vi "Periodic Tasks.vi"(8 "error in":errorcluster) -> ()   [LabVIEW 2018]
doc: "This VI runs in parallel to other tasks. It can contain as many user-defined periodic loops as you need. These can carry out PID or other sorts of timed response."
uses:
  <vilib>/Rock Robotics/WPI/ThirdParty/Phoenix-LabVIEW/Motor Controller/Controls/CTRE_Phoenix_MotorControl_ControlMode.ctl
  <vilib>/Rock Robotics/WPI/Solenoid/WPI_SolenoidValue.ctl
  <vilib>/Rock Robotics/WPI/Utilities/WPI_GetSetVariantRefNum.vi
  Robot Global Data.vi
  <vilib>/Rock Robotics/WPI/Solenoid/WPI_SolenoidSetEnum.vi
  <vilib>/Rock Robotics/WPI/RobotDrive/WPI_RobotDriveArcadeDrive_Standard(NoSaturation).vi
  <vilib>/Rock Robotics/WPI/ThirdParty/Phoenix-LabVIEW/Motor Controller/Get/CTRE_Phoenix_MotorController_GetQuadratureData.vi
panel:
  out "Waveform Chart":T1(graph)
  in  "Zero":bool
  out "Quadrature Position 2":i32
  out "Quadrature Position":i32
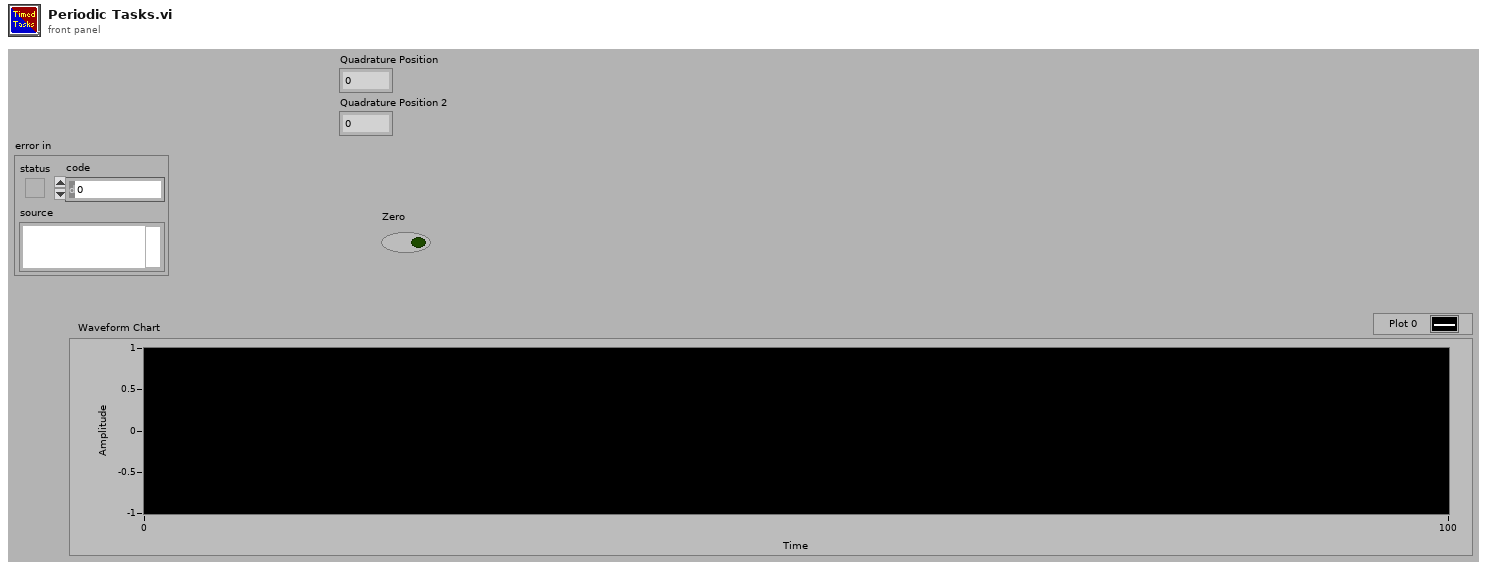
[diagram p1: front panel]
types:
  T1 = cluster{"Quadrature Position":i32, "Quadrature Position":i32}
  T2 = typedef "WPI_MotorControlDeviceRef.ctl" = cluster{"DeviceStatus":errorcluster, "Type":T3, "PWM":cluster{"PWM Channel":T4, "DeadBand":T5}, "CAN":cluster{"Device Number":u8, "SetOutput VI Ref":variant, "GetOutput VI Ref":variant, "Enable VI Ref":variant, "Disable VI Ref":variant, "Data":variant}, "Invert":bool, "DIO PWM":cluster{"PWM \"Enable\" Channel":T4, "DIOChannel":T6, "PWM Rate":dbl}}
  T3 = typedef "WPI_MotorControlType.ctl" = enum16{"PWM", "CAN", "DIO PWM"}
  T4 = typedef "FPGA_DIOPWMChannel.ctl" = enum8{"PWM 0", "PWM 1", "PWM 2", "PWM 3", "PWM 4", "PWM 5", "PWM 6", "PWM 7", "PWM 8", "PWM 9", "PWM MXP 0", "PWM MXP 1", "PWM MXP 2", "PWM MXP 3", "PWM MXP 4", "PWM MXP 5", "PWM MXP 6", "PWM MXP 7", "PWM MXP 8", "PWM MXP 9", "Invalid"}
  T5 = typedef "WPI_PWMDeadband.ctl" = cluster{"Name":string, "maxPositivePwm":i32, "minPositivePwm":i32, "centerPwm":i32, "maxNegativePwm":i32, "minNegativePwm":i32, "angularRange":u16}
  T6 = typedef "FPGA_DIOChannel.ctl" = enum8{"DIO 0", "DIO 1", "DIO 2", "DIO 3", "DIO 4", "DIO 5", "DIO 6", "DIO 7", "DIO 8", "DIO 9", "DIO MXP 0", "DIO MXP 1", "DIO MXP 2", "DIO MXP 3", "DIO MXP 4", "DIO MXP 5", "DIO MXP 6", "DIO MXP 7", "DIO MXP 8", "DIO MXP 9", "DIO MXP 10", "DIO MXP 11", "DIO MXP 12", "DIO MXP 13", "DIO MXP 14", "DIO MXP 15", "SPI Port CS1", "SPI Port CS2", "SPI Port CS3", "SPI Port MISO", "SPI Port MOSI", "Invalid"}
  T7 = typedef "WPI_JoystickDevRef.ctl" = cluster{"Device":T8}
  T8 = typedef "WPI_JoystickDeviceEnum.ctl" = enum16{"USB 0", "USB 1", "USB 2", "USB 3", "USB 4", "USB 5"}
  T9 = typedef "WPI_RobotDriveDevRef.ctl" = cluster{"DevStatus":errorcluster, "Motors[]":T2[], "Square Inputs":bool, "Max Output":dbl}
  T10 = typedef "WPI_SolenoidDevRef.ctl" = cluster{"DevStatus":errorcluster, "Pneumatics Control Module":u8, "Forward Solenoid Channel":T11, "Reverse Solenoid Channel":T11}
  T11 = typedef "WPI_SolenoidChannel.ctl" = enum8{"Solenoid 0", "Solenoid 1", "Solenoid 2", "Solenoid 3", "Solenoid 4", "Solenoid 5", "Solenoid 6", "Solenoid 7", "Invalid"}
  T12 = typedef "WPI_SolenoidValue.ctl" = enum16{"Off", "On", "Forward", "Reverse"}
  T13 = typedef "CTRE_Phoenix_MotorControl_ControlMode.ctl" = u16
  T14 = typedef "WPI_DriverStationRobotMode2.ctl" = enum16{"Autonomous Disabled", "Autonomous Enabled", "Teleop Disabled", "Teleop Enabled", "Disconnected", "Finish", "Test Disabled", "Test Enabled", "Emergency Stopped"}
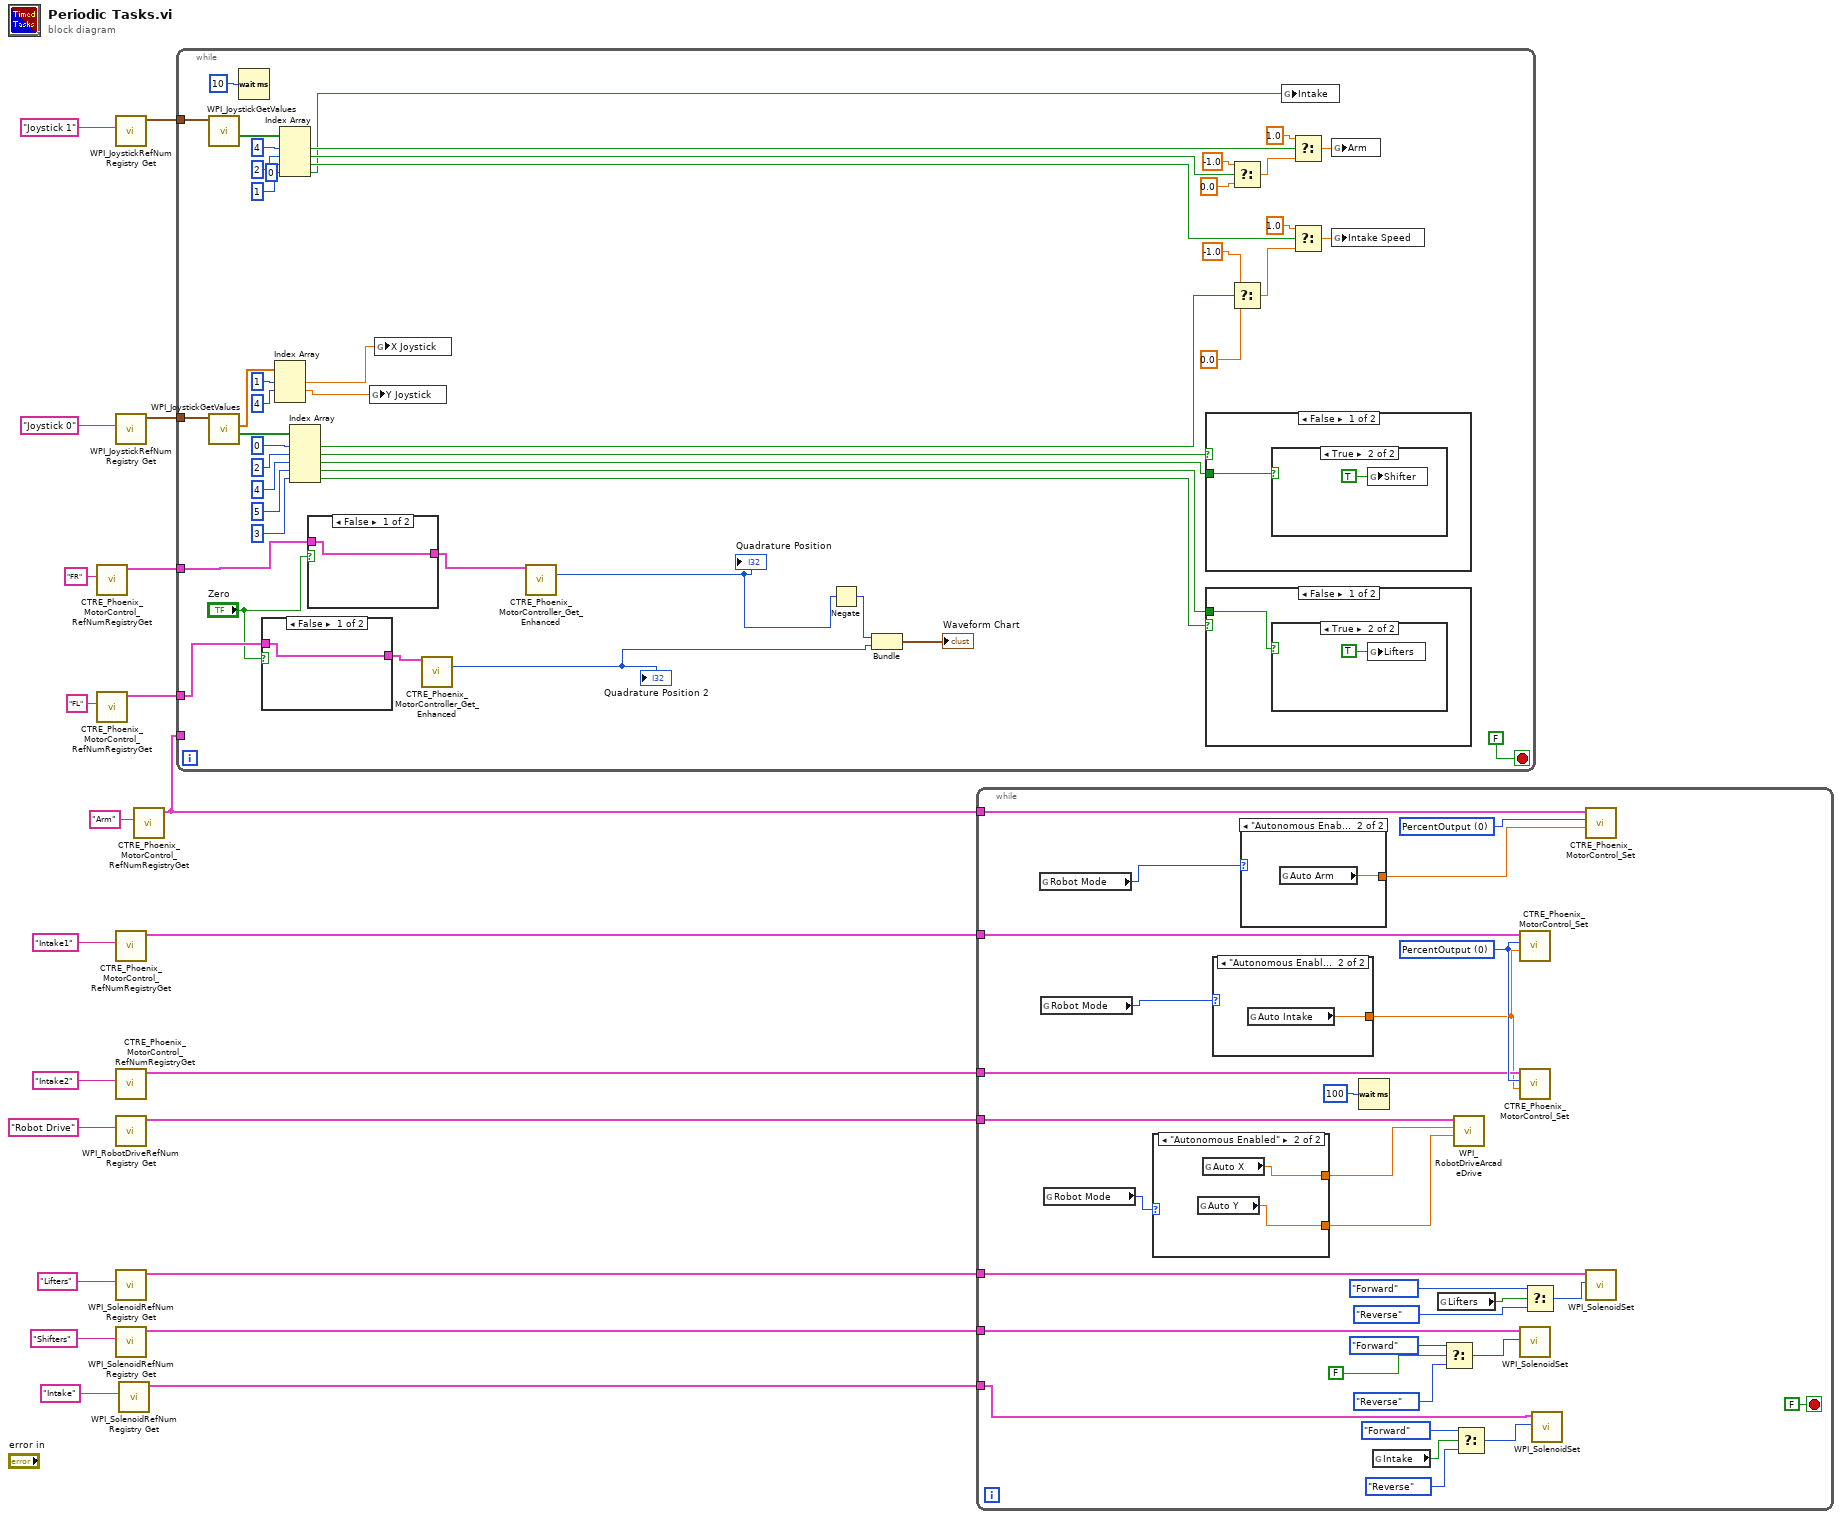
[diagram p0: block diagram]
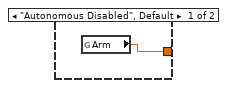
[diagram p2: hidden frame]
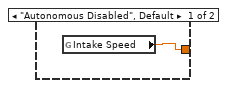
[diagram p3: hidden frame]
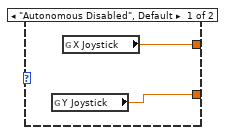
[diagram p4: hidden frame]
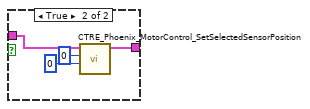
[diagram p5: hidden frame]
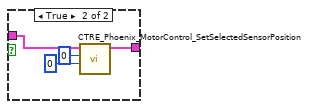
[diagram p6: hidden frame]
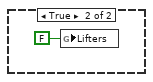
[diagram p8: hidden frame]
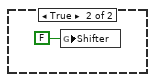
[diagram p10: hidden frame]
diagram:
  n1 = call <vilib>:"CTRE_Phoenix_MotorControl_RefNumRegistryGet.vi"("refnum name"="FR") -> ("PhoenixMotorControlDevRef"=w2:T2)  [unwired: 9 in, 1 out]
  n2 = call <vilib>:"CTRE_Phoenix_MotorControl_RefNumRegistryGet.vi"("refnum name"="FL") -> ("PhoenixMotorControlDevRef"=w1:T2)  [unwired: 9 in, 1 out]
  n3 = call <vilib>:"WPI_JoystickRefNum Registry Get.vi"("refnum name"="Joystick 1") -> ("JoystickDevRef"=w16:T7)  [unwired: 1 in, 9 out]
  n4 = call <vilib>:"WPI_JoystickRefNum Registry Get.vi"("refnum name"="Joystick 0") -> ("JoystickDevRef"=w15:T7)  [unwired: 1 in, 9 out]
  n5 = call <vilib>:"CTRE_Phoenix_MotorControl_RefNumRegistryGet.vi"("refnum name"="Intake1") -> ("PhoenixMotorControlDevRef"=w14:T2)  [unwired: 9 in, 1 out]
  n6 = call <vilib>:"CTRE_Phoenix_MotorControl_RefNumRegistryGet.vi"("refnum name"="Intake2") -> ("PhoenixMotorControlDevRef"=w13:T2)  [unwired: 9 in, 1 out]
  n7 = call <vilib>:"WPI_RobotDriveRefNum Registry Get.vi"("refnum name"="Robot Drive") -> ("RobotDriveDevRef"=w12:T9)  [unwired: 1 in, 9 out]
  n8 = call <vilib>:"WPI_SolenoidRefNum Registry Get.vi"("refnum name"="Lifters") -> ("SolenoidDevRef"=w7:T10)  [unwired: 9 in, 1 out]
  n9 = call <vilib>:"WPI_SolenoidRefNum Registry Get.vi"("refnum name"="Shifters") -> ("SolenoidDevRef"=w9:T10)  [unwired: 9 in, 1 out]
  n10 = call <vilib>:"WPI_SolenoidRefNum Registry Get.vi"("refnum name"="Intake") -> ("SolenoidDevRef"=w5:T10)  [unwired: 9 in, 1 out]
  n11 = call <vilib>:"CTRE_Phoenix_MotorControl_RefNumRegistryGet.vi"("refnum name"="Arm") -> ("PhoenixMotorControlDevRef"=w11:T2)  [unwired: 9 in, 1 out]
  n12 = while {
    tunnel: w16 -> [w55]
    tunnel: w15 -> [w56]
    tunnel: w11 -> [_]
    tunnel: w2 -> [w31]
    tunnel: w1 -> [w33]
    stop <- FALSE stop-if-true
    n13 = call <vilib>:"WPI_JoystickGetValues.vi"("JoystickDevRef"=w55) -> ("Buttons"=w60:bool[])  [unwired: 6 in, 4 out]
    n14 = call <vilib>:"WPI_JoystickGetValues.vi"("JoystickDevRef"=w56) -> ("Buttons"=w59:bool[], "Axes"=w68:dbl[])  [unwired: 6 in, 3 out]
    n15 = Wait (ms)(milliseconds to wait=u32 10) -> ()  [unwired: 1 out]
    n16 = case shown="False" "Zero" {
      tunnel: w33 -> [w76 w80]
      tunnel: [w76 w79] -> w32
      frame False {
      }
      frame True {
        n17 = call <vilib>:"CTRE_Phoenix_MotorControl_SetSelectedSensorPosition.vi"("pidLoopIdx"=u32 0, "New Sensor Position"=0, "PhoenixMotorControlDevRef"=w80) -> ("PhoenixMotorControlDevRef"=w79:T2)  [unwired: 7 in, 1 out]
      }
    }
    n18 = Index Array(array=w68, index #1=1 ("index"), index #2=4 ("index")) -> (element #1=w24:dbl, element #2=w23:dbl)  [unwired: 1 in, 1 out]
    n19 = Index Array(array=w60, index #1=4 ("index"), index #2=2 ("index"), index #3=1 ("index"), index #4=0 ("index")) -> (element #1=w46:bool, element #2=w47:bool, element #3=w52:bool, element #4=w35:bool)
    n20 = Index Array(array=w59, index #1=0 ("index"), index #2=2 ("index"), index #3=4 ("index"), index #4=5 ("index"), index #5=3 ("index")) -> (element #1=w57:bool, element #2=w42:bool, element #3=w41:bool, element #4=w37:bool, element #5=w38:bool)
    n21 = case shown="False" "Zero" {
      tunnel: w31 -> [w71 w75]
      tunnel: [w71 w74] -> w30
      frame False {
      }
      frame True {
        n22 = call <vilib>:"CTRE_Phoenix_MotorControl_SetSelectedSensorPosition.vi"("pidLoopIdx"=u32 0, "New Sensor Position"=0, "PhoenixMotorControlDevRef"=w75) -> ("PhoenixMotorControlDevRef"=w74:T2)  [unwired: 7 in, 1 out]
      }
    }
    n23 = global write "Robot Global Data.vi" "Y Joystick"(w23) -> ()
    n24 = global write "Robot Global Data.vi" "X Joystick"(w24) -> ()
    n25 = call-poly <vilib>:"CTRE_Phoenix_MotorController_Get_Enhanced.vi"("PhoenixMotorControlDevRef"=w32) -> ("Quadrature Position"=w28:i32)  [unwired: 11 in, 3 out]
    "Quadrature Position 2" <- w28
    n26 = call-poly <vilib>:"CTRE_Phoenix_MotorController_Get_Enhanced.vi"("PhoenixMotorControlDevRef"=w30) -> ("Quadrature Position"=w26:i32)  [unwired: 11 in, 3 out]
    "Quadrature Position" <- w26
    n27 = Negate(x=w26) -> (-x=w25:i32)
    n28 = Bundle(w25, "Quadrature Position"=w28) -> (→"Waveform Chart":cluster{i32, "Quadrature Position":i32})  [unwired: 1 in]
    n29 = case shown="False" w42 {
      tunnel: w41 -> [w84 _]
      frame False {
        n30 = case shown="True" w84 {
          frame False {
          }
          frame True {
            n31 = global write "Robot Global Data.vi" "Shifter"(TRUE ("Shifter")) -> ()
          }
        }
      }
      frame True {
        n32 = global write "Robot Global Data.vi" "Shifter"(FALSE ("Shifter")) -> ()
      }
    }
    n33 = case shown="False" w38 {
      tunnel: w37 -> [w81 _]
      frame False {
        n34 = case shown="True" w81 {
          frame False {
          }
          frame True {
            n35 = global write "Robot Global Data.vi" "Lifters"(TRUE ("Shifter")) -> ()
          }
        }
      }
      frame True {
        n36 = global write "Robot Global Data.vi" "Lifters"(FALSE ("Shifter")) -> ()
      }
    }
    n37 = Select(t=-1.0, s=w47, f=0.0) -> (s? t:f=w48:dbl)
    n38 = Select(t=-1.0, s=w57, f=0.0) -> (s? t:f=w63:dbl)
    n39 = global write "Robot Global Data.vi" "Intake"(w35) -> ()
    n40 = Select(t=1.0, s=w46, f=w48) -> (s? t:f=w45:dbl)
    n41 = Select(t=1.0, s=w52, f=w63) -> (s? t:f=w61:dbl)
    n42 = global write "Robot Global Data.vi" "Arm"(w45) -> ()
    n43 = global write "Robot Global Data.vi" "Intake Speed"(w61) -> ()
  }
  n44 = while {
    tunnel: w12 -> [w113]
    tunnel: w11 -> [w109]
    tunnel: w14 -> [w112]
    tunnel: w13 -> [w111]
    tunnel: w9 -> [w108]
    tunnel: w7 -> [w100]
    tunnel: w5 -> [w91]
    stop <- FALSE stop-if-true
    w110 = T13 0 items=["PercentOutput"=0, "Position"=1, "Velocity"=2, "Current"=3, "Follower"=5, "MotionProfile"=6, "MotionMagic"=7, "MotionMagicArc"=8, "MotionProfileArc"=10, "Disabled"=15] ("Control Mode")
    w114 = T13 0 items=["PercentOutput"=0, "Position"=1, "Velocity"=2, "Current"=3, "Follower"=5, "MotionProfile"=6, "MotionMagic"=7, "MotionMagicArc"=8, "MotionProfileArc"=10, "Disabled"=15] ("Control Mode")
    n45 = global read "Robot Global Data.vi" "Robot Mode"() -> (w89:T14)
    n46 = global read "Robot Global Data.vi" "Robot Mode"() -> (w88:T14)
    n47 = global read "Robot Global Data.vi" "Robot Mode"() -> (w90:T14)
    n48 = case shown="\"Autonomous Enabled\"" w90 {
      tunnel: [w122 w123] -> w99
      tunnel: [w121 w124] -> w98
      frame "Autonomous Disabled", Default {
        n49 = global read "Robot Global Data.vi" "Y Joystick"() -> (w122:dbl)
        n50 = global read "Robot Global Data.vi" "X Joystick"() -> (w121:dbl)
      }
      frame "Autonomous Enabled" {
        n51 = global read "Robot Global Data.vi" "Auto Y"() -> (w123:dbl)
        n52 = global read "Robot Global Data.vi" "Auto X"() -> (w124:dbl)
      }
    }
    n53 = case shown="\"Autonomous Enabled\"" w88 {
      tunnel: [w119 w120] -> w97
      frame "Autonomous Disabled", Default {
        n54 = global read "Robot Global Data.vi" "Intake Speed"() -> (w119:dbl)
      }
      frame "Autonomous Enabled" {
        n55 = global read "Robot Global Data.vi" "Auto Intake"() -> (w120:dbl)
      }
    }
    n56 = case shown="\"Autonomous Enabled\"" w89 {
      tunnel: [w117 w118] -> w96
      frame "Autonomous Disabled", Default {
        n57 = global read "Robot Global Data.vi" "Arm"() -> (w117:dbl)
      }
      frame "Autonomous Enabled" {
        n58 = global read "Robot Global Data.vi" "Auto Arm"() -> (w118:dbl)
      }
    }
    n59 = Wait (ms)(milliseconds to wait=u32 100) -> ()  [unwired: 1 out]
    n60 = global read "Robot Global Data.vi" "Intake"() -> (w93:bool)
    n61 = global read "Robot Global Data.vi" "Lifters"() -> (w102:bool)
    n62 = Select(t=WPI_SolenoidValue."Forward" ("Value"), s=FALSE, f=WPI_SolenoidValue."Reverse" ("Value")) -> (s? t:f=w105:T12)
    n63 = call-poly <vilib>:"WPI_RobotDriveArcadeDrive.vi"("Y axis value"=w99, "X axis value"=w98, "RobotDriveDevRef"=w113) -> ()  [unwired: 6 in, 3 out]
    n64 = Select(t=WPI_SolenoidValue."Forward" ("Value"), s=w93, f=WPI_SolenoidValue."Reverse" ("Value")) -> (s? t:f=w92:T12)
    n65 = call <vilib>:"CTRE_Phoenix_MotorControl_Set.vi"("Output"=w97, "Control Mode"=w114, "PhoenixMotorControlDevRef"=w112) -> ()  [unwired: 7 in, 2 out]
    n66 = call <vilib>:"CTRE_Phoenix_MotorControl_Set.vi"("Output"=w97, "Control Mode"=w114, "PhoenixMotorControlDevRef"=w111) -> ()  [unwired: 7 in, 2 out]
    n67 = call-poly <vilib>:"WPI_SolenoidSet.vi"("Value"=w105, "SolenoidDevRef"=w108) -> ()  [unwired: 8 in, 2 out]
    n68 = Select(t=WPI_SolenoidValue."Forward" ("Value"), s=w102, f=WPI_SolenoidValue."Reverse" ("Value")) -> (s? t:f=w101:T12)
    n69 = call-poly <vilib>:"WPI_SolenoidSet.vi"("Value"=w92, "SolenoidDevRef"=w91) -> ()  [unwired: 8 in, 2 out]
    n70 = call <vilib>:"CTRE_Phoenix_MotorControl_Set.vi"("Output"=w96, "Control Mode"=w110, "PhoenixMotorControlDevRef"=w109) -> ()  [unwired: 7 in, 2 out]
    n71 = call-poly <vilib>:"WPI_SolenoidSet.vi"("Value"=w101, "SolenoidDevRef"=w100) -> ()  [unwired: 8 in, 2 out]
  }
